vi "Read Datos Out.vi"(8 "error in (no error)":errorcluster, 11 "Class 2 in":refnum<class "Class 2.lvclass">) -> (0 "error out":errorcluster, 3 "Class 2 out":refnum<class "Class 2.lvclass">)   [LabVIEW 2019, in "Class 2.lvclass"]
uses:
  Class 2.lvclass
  Class 2.lvclass/Class 2.ctl
  Datos Out.vi
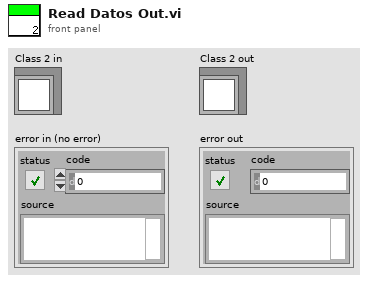
[diagram p1: front panel]
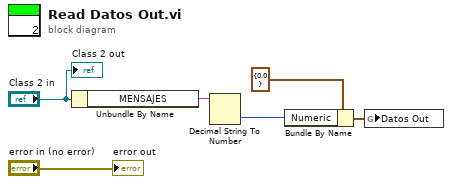
[diagram p0: block diagram]
diagram:
  n1 = Unbundle By Name("Class 2 in") -> ("MENSAJES"=w4:string)
  n2 = Decimal String To Number(string=w4) -> (number=w3:i32)  [unwired: 2 in, 1 out]
  n3 = Bundle By Name(cluster=cluster{"Numeric":dbl} {"Numeric"=0.0} ("Datos Out"), "Numeric"=w3) -> (w2:cluster{"Numeric":dbl})
  n4 = global write "Datos Out.vi" "Datos Out"(w2) -> ()
  "error out" <- "error in (no error)"
  "Class 2 out" <- "Class 2 in"
